vi "Cluster Id FGV.vi"(8 "error in (no error)":errorcluster, 10 "cluster id":string, 11 "action":enum16{"Get Cluster Id", "Set Cluster Id"}(ring)) -> (0 "error out":errorcluster, 3 "cluster id out":string)   [LabVIEW 2021, in "NI Discovery V1 Client.lvlib"]
uses:
  NI Discovery V1 Client.lvlib
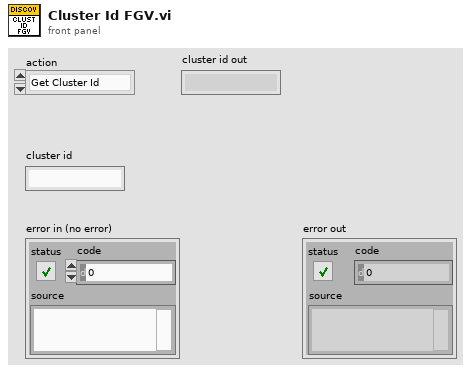
[diagram p1: front panel]
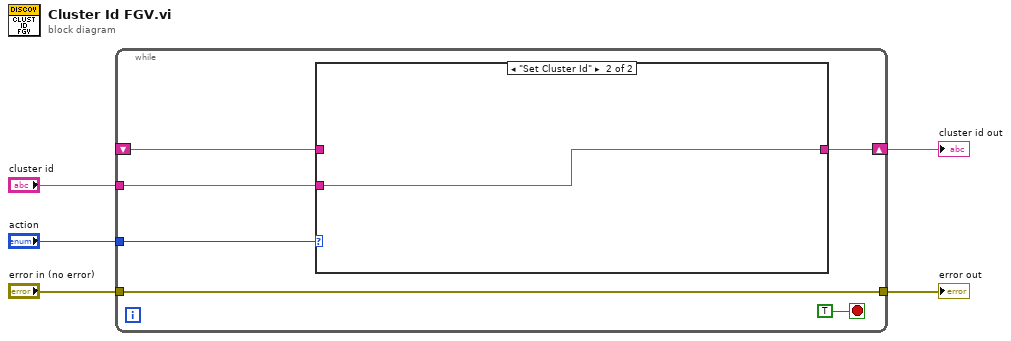
[diagram p0: block diagram]
diagram:
  n1 = while {
    tunnel: "action" -> [w10]
    shift-right: [w8] -> w3
    shift-left: _ -> [w7]
    tunnel: "cluster id" -> [w9]
    tunnel: "error in (no error)" -> [w6]
    tunnel: [w6] -> w1
    stop <- TRUE stop-if-true
    n2 = case shown="\"Set Cluster Id\"" w10 {
      tunnel: w9 -> [_ w13]
      tunnel: [w12 w13] -> w8
      tunnel: w7 -> [w12 _]
      frame "Get Cluster Id", Default {
      }
      frame "Set Cluster Id" {
      }
    }
  }
  "cluster id out" <- w3
  "error out" <- w1
